vi "Write.vi"(7 "Byte Array as Blobs":bool=TRUE, 8 "Error In":errorcluster, 10 "Anything":variant, 11 "Writer In":refnum<class "Writer.lvclass">) -> (0 "Error Out":errorcluster, 3 "Writer Out":refnum<class "Writer.lvclass">)   [LabVIEW 2019, in "LabPack.lvlib"]
doc: "Recursively writes MessagePack data and encodes based on the supplied type."
uses:
  LabPack.lvlib
  Public/Writer/Writer.lvclass
  Public/Writer/Writer.lvclass/Writer.ctl
  <vilib>/Utility/Data Type/Type Definitions/Data Type.ctl
  Public/Writer/Private/Handle Error.vi
  Public/Writer/Public/Status/Read Is Error.vi
  Public/Writer/Public/Status/Read Status.vi
  Public/Writer/Public/Status/Read Status Message.vi
  Public/Writer/Private/Write Nil by Value.vi
  Public/Utility/Status Code.vi
  <vilib>/Utility/error.llb/Error Cluster From Error Code.vi
  Public/Writer/Private/Begin Array by Value.vi
  Public/Writer/Private/End Array by Value.vi
  Public/Writer/Private/Begin Map by Value.vi
  Public/Writer/Private/End Map by Value.vi
  <vilib>/Utility/Data Type/NI_Data Type.lvlib
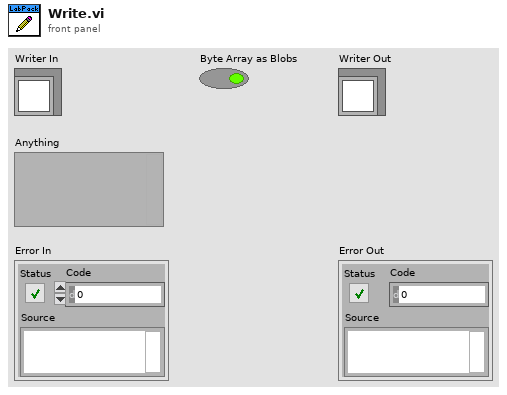
[diagram p1: front panel]
types:
  T1 = typedef "NI_Data Type.lvlib/Data Type.ctl" = enum8{"Invalid Type", "Void", "I8", "I16", "I32", "I64", "U8", "U16", "U32", "U64", "Single Float", "Double Float", "Extended Float", "Single Complex", "Double Complex", "Extended Complex", "Enum U8", "Enum U16", "Enum U32", "Enum U64", "Single Float With Unit", "Double Float With Unit", "Extended Float With Unit", "Single Complex with Unit", "Double Complex with Unit", "Extended Complex with Unit", "Boolean", "String", "Path", "Picture", "Tag", "Array", "Cluster", "Variant", "LV Variant", "Waveform", "Timestamp", "Digital Waveform", "Digital Data", "ExpressData", "Refnum", "External Data", "VI", "Poly VI", "LabVIEW Class Instance", "Fixed Point", "Set Collection", "Map Collection"}
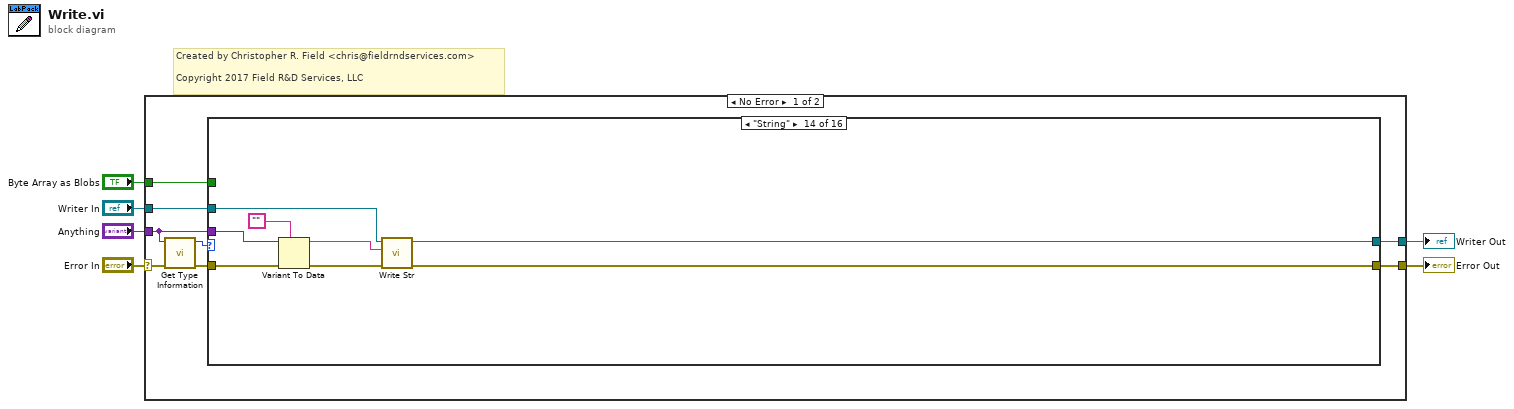
[diagram p0: block diagram]
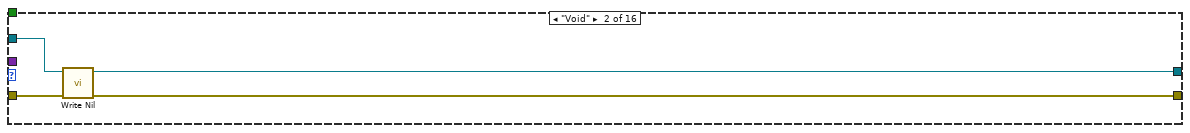
[diagram p3: hidden frame]
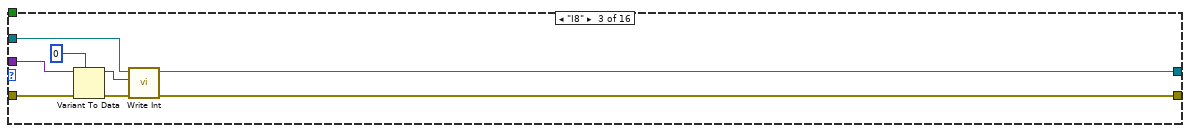
[diagram p4: hidden frame]
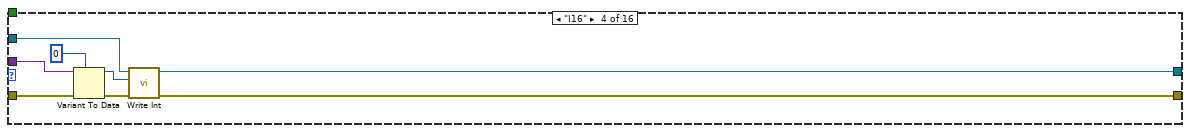
[diagram p5: hidden frame]
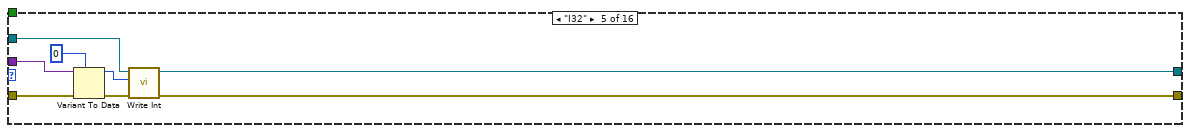
[diagram p6: hidden frame]
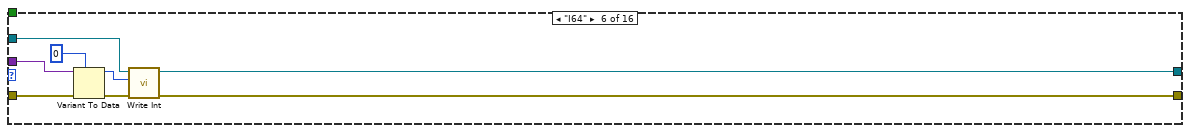
[diagram p7: hidden frame]
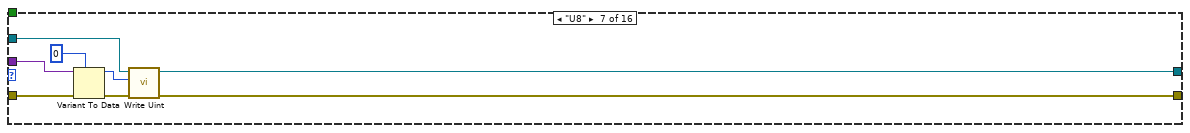
[diagram p8: hidden frame]
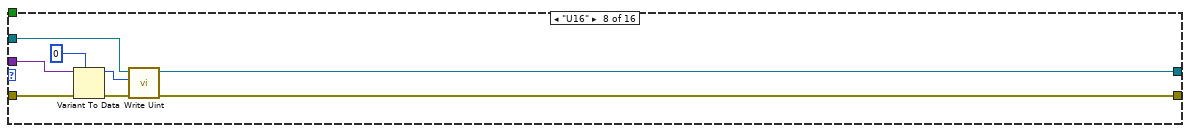
[diagram p9: hidden frame]
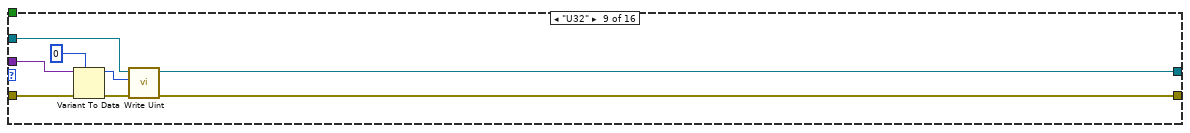
[diagram p10: hidden frame]
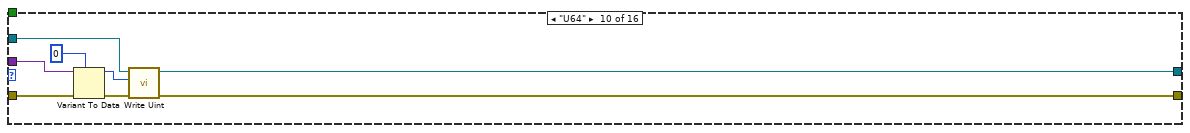
[diagram p11: hidden frame]
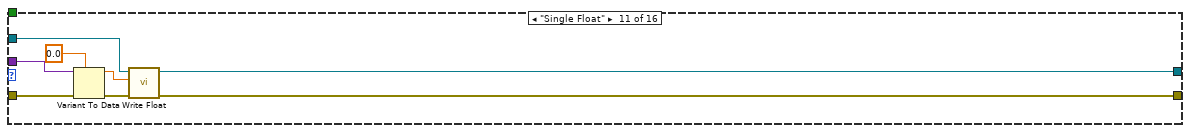
[diagram p12: hidden frame]
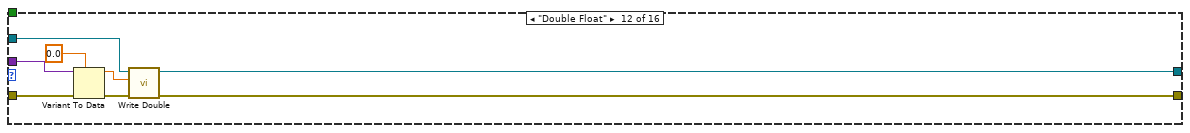
[diagram p13: hidden frame]
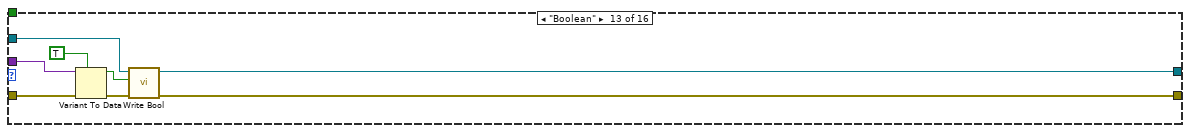
[diagram p14: hidden frame]
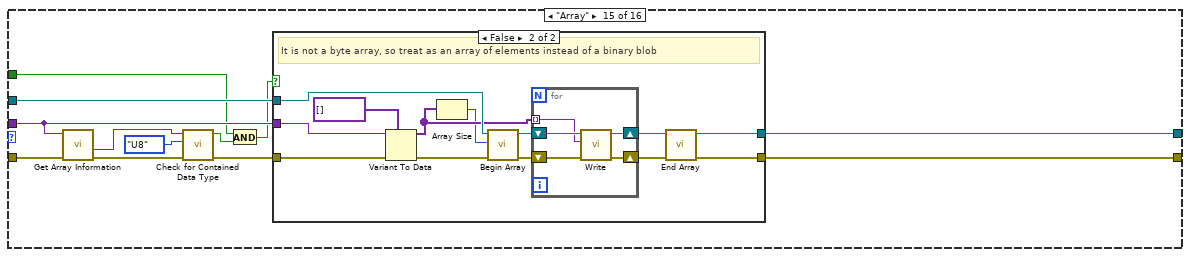
[diagram p15: hidden frame]
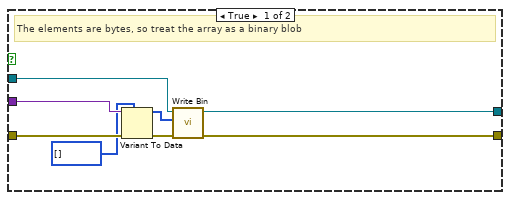
[diagram p16: hidden frame]
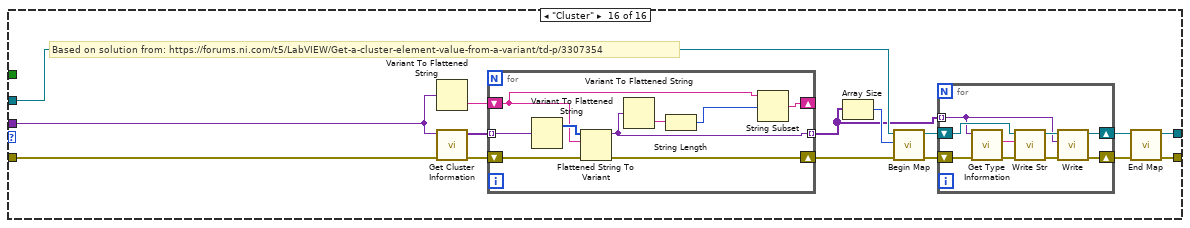
[diagram p17: hidden frame]
diagram:
  # "Created by Christopher R. Field <chris@fieldrndservices.com>\n\nCopyright 2017 Field R&D Services, LLC"
  n1 = case shown="No Error" "Error In" {
    selector: "Error In" -> [w8 w188]
    tunnel: "Anything" -> [w14 _]
    tunnel: "Writer In" -> [w13 w189]
    tunnel: [w12 w189] -> w4
    tunnel: [w11 w188] -> w3
    tunnel: "Byte Array as Blobs" -> [w7 _]
    frame No Error {
      n2 = call <vilib>:"Get Type Information.vi"("error in (no error)"=w8, "variant"=w14) -> ("error out"=w10:errorcluster, "type"=w9:T1)  [unwired: 5 in, 3 out]
      n3 = case shown="\"String\"" w9 {
        tunnel: w10 -> [w15 w18 w28 w36 w44 w52 w60 w68 w76 w84 w92 w100 w106 w116 w124 w161]
        tunnel: [w15 w17 w22 w30 w38 w46 w54 w62 w70 w78 w86 w94 w105 w111 w126 w167] -> w11
        tunnel: [w16 w19 w24 w32 w40 w48 w56 w64 w72 w80 w88 w96 w107 w113 w127 w168] -> w12
        tunnel: w13 -> [w16 w20 w27 w35 w43 w51 w59 w67 w75 w83 w91 w99 w108 w115 w128 w169]
        tunnel: w14 -> [_ _ w26 w34 w42 w50 w58 w66 w74 w82 w90 w98 w103 w114 w125 w160]
        tunnel: w7 -> [_ _ _ _ _ _ _ _ _ _ _ _ _ _ w117 _]
        frame "Invalid Type", Default {
        }
        frame "Void" {
          n4 = call-poly "Write Nil.vi"("Error In"=w18, "Writer In"=w20) -> ("Error Out"=w17:errorcluster, "Writer Out"=w19:refnum<class "Writer.lvclass">)  [unwired: 8 in]
        }
        frame "I8" {
          n5 = Variant To Data(error in=w28, type=i8 0, Variant=w26) -> (data=w21:i8, error out=w23:errorcluster)
          n6 = call "Write Int.vi"("Error In"=w23, "Value"=w21, "Writer In"=w27) -> ("Error Out"=w22:errorcluster, "Writer Out"=w24:refnum<class "Writer.lvclass">)  [unwired: 7 in]
        }
        frame "I16" {
          n7 = Variant To Data(error in=w36, type=i16 0, Variant=w34) -> (data=w29:i16, error out=w31:errorcluster)
          n8 = call "Write Int.vi"("Error In"=w31, "Value"=w29, "Writer In"=w35) -> ("Error Out"=w30:errorcluster, "Writer Out"=w32:refnum<class "Writer.lvclass">)  [unwired: 7 in]
        }
        frame "I32" {
          n9 = Variant To Data(error in=w44, type=0, Variant=w42) -> (data=w37:i32, error out=w39:errorcluster)
          n10 = call "Write Int.vi"("Error In"=w39, "Value"=w37, "Writer In"=w43) -> ("Error Out"=w38:errorcluster, "Writer Out"=w40:refnum<class "Writer.lvclass">)  [unwired: 7 in]
        }
        frame "I64" {
          n11 = Variant To Data(error in=w52, type=i64 0, Variant=w50) -> (data=w45:i64, error out=w47:errorcluster)
          n12 = call "Write Int.vi"("Error In"=w47, "Value"=w45, "Writer In"=w51) -> ("Error Out"=w46:errorcluster, "Writer Out"=w48:refnum<class "Writer.lvclass">)  [unwired: 7 in]
        }
        frame "U8" {
          n13 = Variant To Data(error in=w60, type=u8 0, Variant=w58) -> (data=w53:u8, error out=w55:errorcluster)
          n14 = call "Write Uint.vi"("Error In"=w55, "Value"=w53, "Writer In"=w59) -> ("Error Out"=w54:errorcluster, "Writer Out"=w56:refnum<class "Writer.lvclass">)  [unwired: 7 in]
        }
        frame "U16" {
          n15 = Variant To Data(error in=w68, type=u16 0, Variant=w66) -> (data=w61:u16, error out=w63:errorcluster)
          n16 = call "Write Uint.vi"("Error In"=w63, "Value"=w61, "Writer In"=w67) -> ("Error Out"=w62:errorcluster, "Writer Out"=w64:refnum<class "Writer.lvclass">)  [unwired: 7 in]
        }
        frame "U32" {
          n17 = Variant To Data(error in=w76, type=u32 0, Variant=w74) -> (data=w69:u32, error out=w71:errorcluster)
          n18 = call "Write Uint.vi"("Error In"=w71, "Value"=w69, "Writer In"=w75) -> ("Error Out"=w70:errorcluster, "Writer Out"=w72:refnum<class "Writer.lvclass">)  [unwired: 7 in]
        }
        frame "U64" {
          n19 = Variant To Data(error in=w84, type=u64 0, Variant=w82) -> (data=w77:u64, error out=w79:errorcluster)
          n20 = call "Write Uint.vi"("Error In"=w79, "Value"=w77, "Writer In"=w83) -> ("Error Out"=w78:errorcluster, "Writer Out"=w80:refnum<class "Writer.lvclass">)  [unwired: 7 in]
        }
        frame "Single Float" {
          n21 = Variant To Data(error in=w92, type=sgl 0.0, Variant=w90) -> (data=w85:sgl, error out=w87:errorcluster)
          n22 = call "Write Float.vi"("Error In"=w87, "Value"=w85, "Writer In"=w91) -> ("Error Out"=w86:errorcluster, "Writer Out"=w88:refnum<class "Writer.lvclass">)  [unwired: 7 in]
        }
        frame "Double Float" {
          n23 = Variant To Data(error in=w100, type=0.0, Variant=w98) -> (data=w93:dbl, error out=w95:errorcluster)
          n24 = call "Write Double.vi"("Error In"=w95, "Value"=w93, "Writer In"=w99) -> ("Error Out"=w94:errorcluster, "Writer Out"=w96:refnum<class "Writer.lvclass">)  [unwired: 7 in]
        }
        frame "Boolean" {
          n25 = Variant To Data(error in=w106, type=TRUE, Variant=w103) -> (data=w101:bool, error out=w104:errorcluster)
          n26 = call "Write Bool.vi"("Error In"=w104, "Value"=w101, "Writer In"=w108) -> ("Error Out"=w105:errorcluster, "Writer Out"=w107:refnum<class "Writer.lvclass">)  [unwired: 7 in]
        }
        frame "String" {
          n27 = Variant To Data(error in=w116, type="", Variant=w114) -> (data=w109:string, error out=w112:errorcluster)
          n28 = call "Write Str.vi"("Error In"=w112, "Value"=w109, "Writer In"=w115) -> ("Error Out"=w111:errorcluster, "Writer Out"=w113:refnum<class "Writer.lvclass">)  [unwired: 7 in]
        }
        frame "Array" {
          n29 = call <vilib>:"Get Array Information.vi"("error in (no error)"=w124, "variant"=w125) -> ("error out"=w122:errorcluster, "array element data type"=w123:variant)  [unwired: 6 in, 2 out]
          n30 = call <vilib>:"Check for Contained Data Type.vi"("error in (no error)"=w122, "data type to find"=Data_Type."U8" ("Data Type to Find"), "variant"=w123) -> ("error out"=w120:errorcluster, "contains data type to find?"=w119:bool)  [unwired: 7 in]
          n31 = And(x=w117, y=w119) -> (x .and. y?=w118:bool)
          n32 = case shown="False" w118 {
            tunnel: w128 -> [w136 w149]
            tunnel: [w135 w148] -> w127
            tunnel: [w129 w147] -> w126
            tunnel: w125 -> [w133 w138]
            tunnel: w120 -> [w134 w137]
            frame True {
              # "The elements are bytes, so treat the array as a binary blob"
              n33 = Variant To Data(error in=w134, type=u8[] [], Variant=w133) -> (data=w131:u8[], error out=w130:errorcluster)
              n34 = call "Write Bin.vi"("Error In"=w130, "Value"=w131, "Writer In"=w136) -> ("Error Out"=w129:errorcluster, "Writer Out"=w135:refnum<class "Writer.lvclass">)  [unwired: 7 in]
            }
            frame False {
              # "It is not a byte array, so treat as an array of elements instead of a binary blob"
              n35 = Variant To Data(error in=w137, type=variant[] [], Variant=w138) -> (data=w140:variant[], error out=w142:errorcluster)
              n36 = Array Size(array=w140) -> (size(s)=w139:i32)
              n37 = call-poly "Begin Array.vi"("Error In"=w142, "Elements Count"=w139, "Writer In"=w149) -> ("Error Out"=w143:errorcluster, "Writer Out"=w146:refnum<class "Writer.lvclass">)  [unwired: 7 in]
              n38 = for {
                shift-right: [w153] -> w145
                shift-left: w146 -> [w154]
                shift-right: [w152] -> w144
                shift-left: w143 -> [w151]
                tunnel: w140 -> [w150] mode=indexing
                n39 = call "Write.vi"("Error In"=w151, "Anything"=w150, "Writer In"=w154) -> ("Error Out"=w152:errorcluster, "Writer Out"=w153:refnum<class "Writer.lvclass">)  [unwired: 7 in]
              }
              n40 = call-poly "End Array.vi"("Error In"=w144, "Writer In"=w145) -> ("Error Out"=w147:errorcluster, "Writer Out"=w148:refnum<class "Writer.lvclass">)  [unwired: 8 in]
            }
          }
        }
        frame "Cluster" {
          # "Based on solution from: https://forums.ni.com/t5/LabVIEW/Get-a-cluster-element-value-from-a-variant/td-p/3307354"
          n41 = Variant To Flattened String(Variant=w160) -> (data string=w159:string)  [unwired: 1 out]
          n42 = call <vilib>:"Get Cluster Information.vi"("error in (no error)"=w161, "variant"=w160) -> ("error out"=w157:errorcluster, "cluster elements"=w158:variant[])  [unwired: 8 in]
          n43 = for {
            shift-right: [w178] -> _
            shift-left: w159 -> [w173]
            tunnel: w158 -> [w175] mode=indexing
            shift-right: [w171] -> w156
            shift-left: w157 -> [w172]
            tunnel: [w170] -> w155 mode=indexing
            n44 = Variant To Flattened String(Variant=w175) -> (1:w174:i16[])  [unwired: 1 out]
            n45 = Flattened String To Variant(4:w172, 6:w173, 7:w174) -> (0:w171:errorcluster, 3:w170:variant)
            n46 = Variant To Flattened String(Variant=w170) -> (data string=w176:string)  [unwired: 1 out]
            n47 = String Length(string=w176) -> (length=w177:i32)
            n48 = String Subset(string=w173, offset (0)=w177) -> (substring=w178:string)  [unwired: 1 in]
          }
          n49 = Array Size(array=w155) -> (size(s)=w162:i32)
          n50 = call-poly "Begin Map.vi"("Error In"=w156, "Elements Count"=w162, "Writer In"=w169) -> ("Error Out"=w163:errorcluster, "Writer Out"=w166:refnum<class "Writer.lvclass">)  [unwired: 7 in]
          n51 = for {
            shift-right: [w186] -> w165
            shift-left: w166 -> [w187]
            shift-right: [w185] -> w164
            shift-left: w163 -> [w184]
            tunnel: w155 -> [w179] mode=indexing
            n52 = call <vilib>:"Get Type Information.vi"("error in (no error)"=w184, "variant"=w179) -> ("error out"=w182:errorcluster, "name"=w180:string)  [unwired: 5 in, 3 out]
            n53 = call "Write Str.vi"("Error In"=w182, "Value"=w180, "Writer In"=w187) -> ("Error Out"=w181:errorcluster, "Writer Out"=w183:refnum<class "Writer.lvclass">)  [unwired: 7 in]
            n54 = call "Write.vi"("Error In"=w181, "Anything"=w179, "Writer In"=w183) -> ("Error Out"=w185:errorcluster, "Writer Out"=w186:refnum<class "Writer.lvclass">)  [unwired: 7 in]
          }
          n55 = call-poly "End Map.vi"("Error In"=w164, "Writer In"=w165) -> ("Error Out"=w167:errorcluster, "Writer Out"=w168:refnum<class "Writer.lvclass">)  [unwired: 8 in]
        }
      }
    }
    frame Error {
    }
  }
  "Writer Out" <- w4
  "Error Out" <- w3
